vi "zmq_z85_encode.vi"(3 "error in":errorcluster, 4 "zero pad? (F)":bool, 5 "data in":u8[](array[numeric])) -> (0 "error out":errorcluster, 2 "encoded string":string)   [LabVIEW 2025, in "ZeroMQ.lvlib"]
doc: "Queries and returns the version of ZeroMQ currently loaded as both a string and struct.\n\nDetailed API documentation: http://api.zeromq.org/3-2:zmq-version"
uses:
  ZeroMQ.lvlib
panel:
  # "ØMQ"
  # "labview"
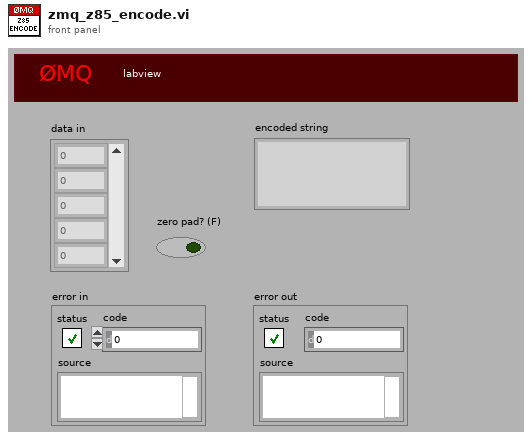
[diagram p1: front panel]
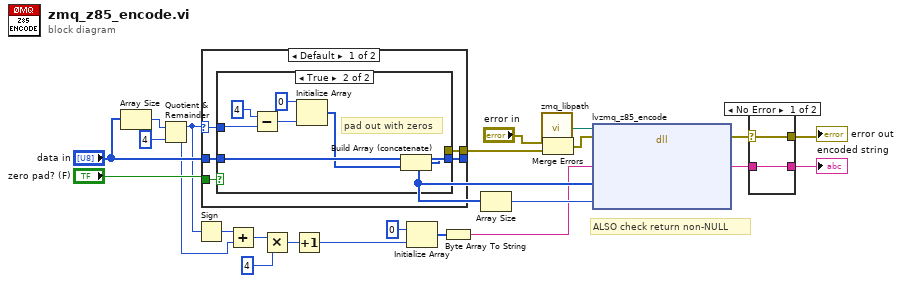
[diagram p0: block diagram]
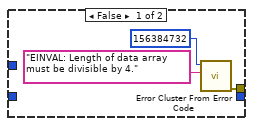
[diagram p3: hidden frame]
diagram:
  # "ALSO check return non-NULL"
  n1 = Array Size(array="data in") -> (size(s)=w11:i32)
  n2 = Quotient & Remainder(x=w11, y=4) -> (x-y*floor(x/y)=w10:i32, floor(x/y)=w8:i32)
  n3 = Sign(1:w10) -> (0:w9:i32)
  n4 = case shown="Default" w10 {
    selector: w10 -> [w27 _]
    tunnel: "zero pad? (F)" -> [w29 _]
    tunnel: "data in" -> [w28 w40]
    tunnel: [w26 w40] -> w19
    tunnel: [w25 _] -> w15
    frame Default {
      n5 = case shown="True" w29 {
        tunnel: w28 -> [_ w37]
        tunnel: w27 -> [_ w39]
        tunnel: [_ w33] -> w26
        tunnel: [w30 _] -> w25
        frame False {
          n6 = call <vilib>:"Error Cluster From Error Code.vi"("error message (\"\")"="EINVAL: Length of data array must be divisible by 4." ("error message (\"\")"), "error code (0)"=156384732) -> ("error out"=w30:errorcluster)  [unwired: 7 in]
        }
        frame True {
          # "pad out with zeros"
          n7 = Subtract(x=4 ("y"), y=w39) -> (x-y=w36:i32)
          n8 = Initialize Array(u8 0 ("element"), w36) -> (w34:u8[])
          n9 = Build Array (concatenate)(w37, w34) -> (w33:u8[])
        }
      }
    }
    frame 0 {
      # "Divisible by 4, is ok"
    }
  }
  n10 = Add(x=w9, y=w8) -> (x+y=w7:i32)
  n11 = Multiply(x=w7, y=4) -> (x*y=w5:i32)
  n12 = Increment(x=w5) -> (x+1=w12:i32)
  n13 = Initialize Array(u8 0 ("element"), w12) -> (w14:u8[])
  n14 = Byte Array To String(unsigned byte array=w14) -> (string=w13:string)
  n15 = Array Size(array=w19) -> (size(s)=w18:i32)
  n16 = call "zmq_libpath.vi"() -> ("path"=w24:path)
  n17 = Merge Errors("error in", w15) -> (w17:errorcluster)
  n18 = dll-call lib="?" fn="lvzmq_z85_encode" ("zmq_labview.dll:lvzmq_socket")(path in=w24, error in=w17, "dest"=w13, "src"=w19, "len"=w18) -> (error out=w4:errorcluster, "dest"=w1:string)  [unwired: 4 in, 1 out]
  n19 = case shown="No Error" w4 {
    selector: w4 -> [w42 w43]
    tunnel: [w42 w43] -> w3
    tunnel: [w41 _] -> w2
    tunnel: w1 -> [w41 _]
    frame No Error {
    }
    frame Error {
    }
  }
  "error out" <- w3
  "encoded string" <- w2
